vi "iq to iq cluster.vi"(0 "i in":fxp<+/-,64,1> format="%.64g", 5 "q in":fxp<+/-,64,1> format="%.64g") -> (4 "data out":T1)   [LabVIEW 2018]
uses:
  <instrlib>/_niInstr/DSP/v1/Shared/Public/IQ Data.ctl
  <instrlib>/_niInstr/DSP/v1/Shared/niInstr DSP v1 Shared.lvlib
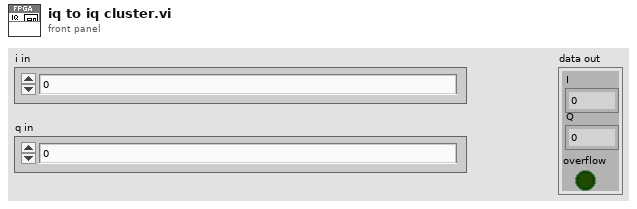
[diagram p1: front panel]
types:
  T1 = typedef "niInstr DSP v1 Shared.lvlib/IQ Data.ctl" = cluster{"I":fxp<+/-,18,1>, "Q":fxp<+/-,18,1>, "overflow":bool}
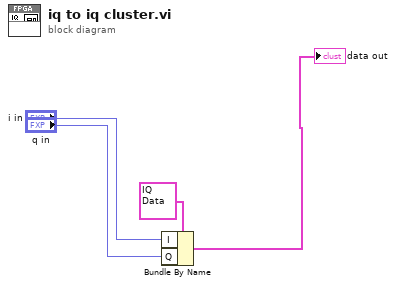
[diagram p0: block diagram]
diagram:
  n1 = Bundle By Name(cluster=T1 {"I"=0.0, "Q"=0.0, "overflow"=FALSE} ("data out"), "I"="i in", "Q"="q in") -> (→"data out":T1)
